vi "sv_Compute Time to Next Optimum for Square Wave.vi"(7 "optimum":T1, 9 "duty cycle (50 %)":dbl=50.0, 10 "phase (0 °)":dbl, 11 "frequency (997 Hz)":dbl=997.0) -> (3 "time to optimum [s]":dbl)   [LabVIEW 2017, in "SoundVib_Generation.lvlib"]
uses:
  <vilib>/addons/_NISVFA/_Generation/SoundVib_Generation.lvlib
  <vilib>/addons/_NISVFA/_Generation/subVIs/sv_Optimum Location.ctl
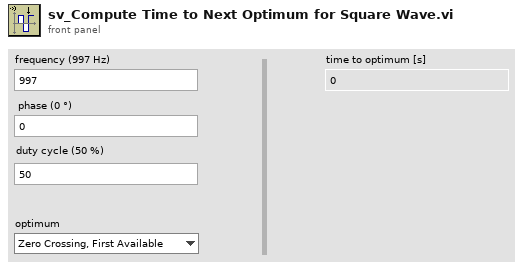
[diagram p1: front panel]
types:
  T1 = typedef "SoundVib_Generation.lvlib/sv_Optimum Location.ctl" = enum16{"Zero Crossing, First Available", "Zero Crossing, Positive Slope", "Zero Crossing, Negative Slope", "Peak or Valley", "Peak", "Valley"}
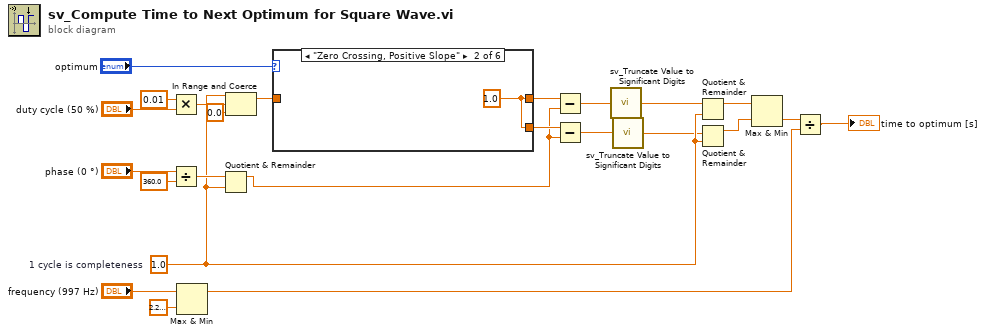
[diagram p0: block diagram]
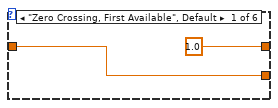
[diagram p2: hidden frame]
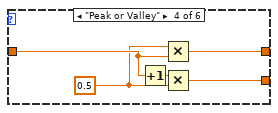
[diagram p4: hidden frame]
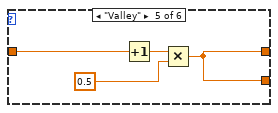
[diagram p5: hidden frame]
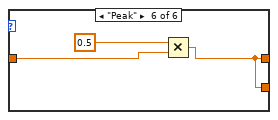
[diagram p6: hidden frame]
diagram:
  w7 = 1.0  # 1 cycle is completeness
  n1 = Multiply(x=0.01, y="duty cycle (50 %)") -> (x*y=w8:dbl)
  n2 = Divide(x="phase (0 °)", y=360.0 ("time to optimum [s]")) -> (x/y=w21:dbl)
  n3 = Max & Min(x="frequency (997 Hz)", y=2.220446049250313e-16) -> (max(x,y)=w13:dbl)  [unwired: 1 out]
  n4 = Quotient & Remainder(x=w21, y=w7) -> (x-y*floor(x/y)=w6:dbl)  [unwired: 1 out]
  n5 = In Range and Coerce(upper limit=w7, x=w8, lower limit=0.0) -> (coerced(x)=w9:dbl)  [unwired: 1 out]
  n6 = case shown="\"Zero Crossing, Positive Slope\"" "optimum" {
    tunnel: [1.0 ("time to optimum [s]") w27 w28 w33 w34 w38] -> w12
    tunnel: [w25 w27 w28 w29 w34 w38] -> w11
    tunnel: w9 -> [w25 _ w28 w32 w37 w40]
    frame "Zero Crossing, First Available", Default {
    }
    frame "Zero Crossing, Positive Slope" {
      w27 = 1.0 ("time to optimum [s]")
    }
    frame "Zero Crossing, Negative Slope" {
    }
    frame "Peak or Valley" {
      w30 = 0.5 ("x")
      n7 = Increment(x=w32) -> (x+1=w31:dbl)
      n8 = Multiply(x=w30, y=w32) -> (x*y=w33:dbl)
      n9 = Multiply(x=w31, y=w30) -> (x*y=w29:dbl)
    }
    frame "Valley" {
      n10 = Increment(x=w37) -> (x+1=w36:dbl)
      n11 = Multiply(x=w36, y=0.5 ("x")) -> (x*y=w34:dbl)
    }
    frame "Peak" {
      n12 = Multiply(x=0.5, y=w40) -> (x*y=w38:dbl)
    }
  }
  n13 = Subtract(x=w12, y=w6) -> (x-y=w2:dbl)
  n14 = Subtract(x=w11, y=w6) -> (x-y=w4:dbl)
  n15 = call <vilib>:"sv_Truncate Value to Significant Digits.vi"("value"=w2) -> ("truncated value"=w1:dbl)  [unwired: 14 in]
  n16 = call <vilib>:"sv_Truncate Value to Significant Digits.vi"("value"=w4) -> ("truncated value"=w3:dbl)  [unwired: 14 in]
  n17 = Quotient & Remainder(x=w1, y=w7) -> (x-y*floor(x/y)=w20:dbl)  [unwired: 1 out]
  n18 = Quotient & Remainder(x=w3, y=w7) -> (x-y*floor(x/y)=w19:dbl)  [unwired: 1 out]
  n19 = Max & Min(x=w20, y=w19) -> (min(x,y)=w18:dbl)  [unwired: 1 out]
  n20 = Divide(x=w18, y=w13) -> (x/y=→"time to optimum [s]":dbl)
